vi "Create_Device.vi"(8 "error in (no error)":errorcluster, 11 "USB-87Pn_Data In":T1) -> (0 "error out":errorcluster, 3 "USB-87Pn_Data Out":T1)   [LabVIEW 2019, in "USB-87P8_Manager.lvlib"]
uses:
  Module/USB-87P8_Manager.lvlib
  USB-87Pn_Data.ctl
  USB-87Pn.lvclass
  Module/DO_Module_Data.ctl
  Module/Module_Data.ctl
  Module/AI_Module_Data.ctl
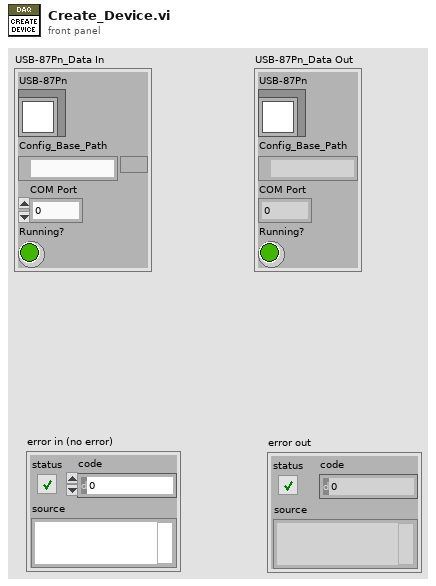
[diagram p1: front panel]
types:
  T1 = typedef "USB-87P8_Manager.lvlib/USB-87Pn_Data.ctl" = cluster{"USB-87Pn":refnum<class "USB-87Pn.lvclass">, "Config_Base_Path":path, "COM Port":i32, "Running?":bool}
  T2 = typedef "USB-87Pn.lvlib/USB-87Pn.lvclass/AI_Module_Data.ctl" = cluster{"Module_Data":T3, "AI_Channels":cluster{"Enabled":bool, "Alias":string}[]}
  T3 = typedef "USB-87Pn.lvlib/USB-87Pn.lvclass/Module_Data.ctl" = cluster{"Number of Channels":u8, "Address":i16, "Alias":string}
  T4 = typedef "USB-87Pn.lvlib/USB-87Pn.lvclass/DO_Module_Data.ctl" = cluster{"Module_Data":T3, "DO_Channels":cluster{"Enabled":bool, "Alias":string}[]}
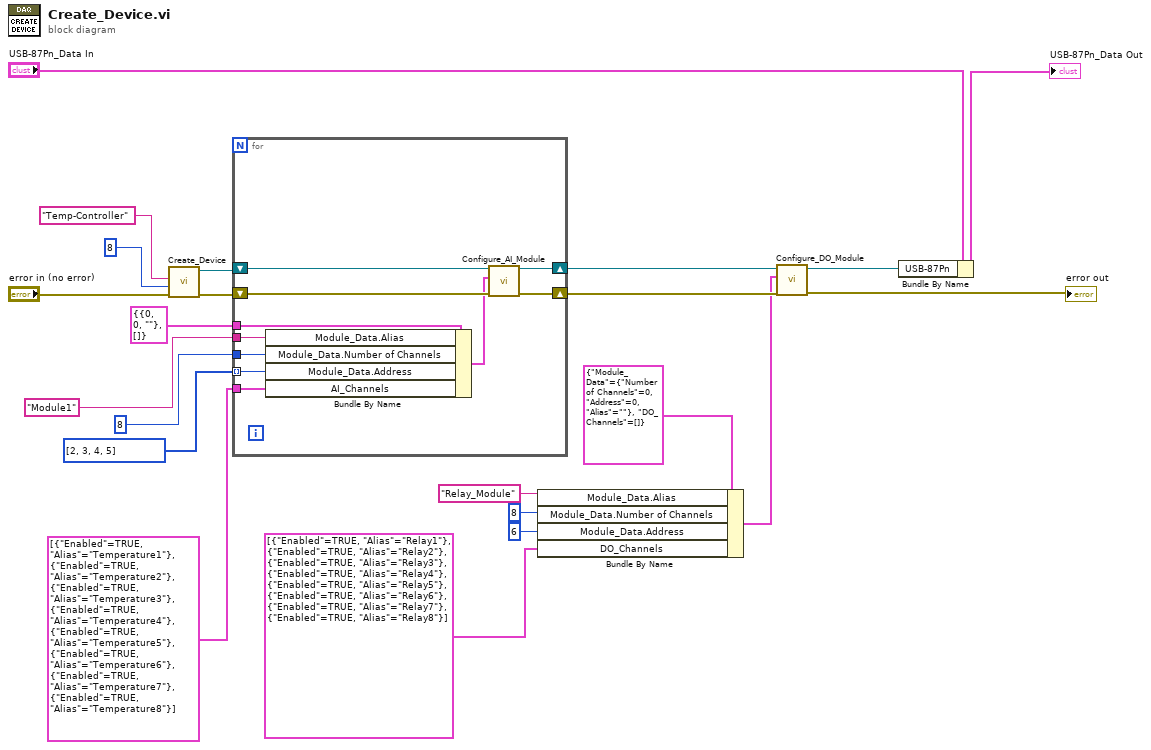
[diagram p0: block diagram]
diagram:
  n1 = call "Create_Device.vi"("error in (no error)"="error in (no error)", "Number of Slots"=i8 8, "Device Name"="Temp-Controller") -> ("error out"=w20:errorcluster, "87Pn out"=w21:refnum<class "USB-87Pn.lvclass">)  [unwired: 7 in]
  n2 = for {
    shift-right: [w30] -> w19
    shift-left: w21 -> [w31]
    shift-right: [w29] -> w18
    shift-left: w20 -> [w32]
    tunnel: T2 {"Module_Data"={"Number of Channels"=0, "Address"=0, "Alias"=""}, "AI_Channels"=[]} ("AI_Module_Data") -> [w28]
    tunnel: "Module1" ("Module_Data.Alias") -> [w27]
    tunnel: u8 8 ("Module_Data.Number of Channels") -> [w26]
    tunnel: cluster{"Enabled":bool, "Alias":string}[] [{"Enabled"=TRUE, "Alias"="Temperature1"}, {"Enabled"=TRUE, "Alias"="Temperature2"}, {"Enabled"=TRUE, "Alias"="Temperature3"}, {"Enabled"=TRUE, "Alias"="Temperature4"}, {"Enabled"=TRUE, "Alias"="Temperature5"}, {"Enabled"=TRUE, "Alias"="Temperature6"}, {"Enabled"=TRUE, "Alias"="Temperature7"}, {"Enabled"=TRUE, "Alias"="Temperature8"}] ("AI_Channels") -> [w25]
    tunnel: i16[] [2, 3, 4, 5] -> [w23] mode=indexing
    n3 = Bundle By Name(cluster=w28, "Module_Data.Alias"=w27, "Module_Data.Number of Channels"=w26, "Module_Data.Address"=w23, "AI_Channels"=w25) -> (w24:T2)
    n4 = call "Configure_AI_Module.vi"("error in (no error)"=w32, "AI_Module_Data"=w24, "USB-87Pn"=w31) -> ("error out"=w29:errorcluster, "USB-87Pn"=w30:refnum<class "USB-87Pn.lvclass">)  [unwired: 7 in]
  }
  n5 = Bundle By Name(cluster=T4 {"Module_Data"={"Number of Channels"=0, "Address"=0, "Alias"=""}, "DO_Channels"=[]} ("DO_Module_Data"), "Module_Data.Alias"="Relay_Module", "Module_Data.Number of Channels"=u8 8, "Module_Data.Address"=i16 6, "DO_Channels"=cluster{"Enabled":bool, "Alias":string}[] [{"Enabled"=TRUE, "Alias"="Relay1"}, {"Enabled"=TRUE, "Alias"="Relay2"}, {"Enabled"=TRUE, "Alias"="Relay3"}, {"Enabled"=TRUE, "Alias"="Relay4"}, {"Enabled"=TRUE, "Alias"="Relay5"}, {"Enabled"=TRUE, "Alias"="Relay6"}, {"Enabled"=TRUE, "Alias"="Relay7"}, {"Enabled"=TRUE, "Alias"="Relay8"}]) -> (w12:T4)
  n6 = call "Configure_DO_Module.vi"("error in (no error)"=w18, "DO_Module_Data"=w12, "USB-87Pn in"=w19) -> ("error out"=→"error out":errorcluster, "USB-87Pn out"=w1:refnum<class "USB-87Pn.lvclass">)  [unwired: 7 in]
  n7 = Bundle By Name(cluster="USB-87Pn_Data In", "USB-87Pn"=w1) -> (→"USB-87Pn_Data Out":T1)
